vi "PinholesRolling.vi"(4 "Current Threshold [nA]":dbl, 5 "settling\ndelay":i32) -> (1 "excluded channels":i32[](array[numeric]), 2 "Current [nA]":dbl[](array[numeric]), 3 "Flag":i32[](array[numeric]))   [LabVIEW 2019]
uses:
  general_VIs/globals/QC_MeasurementSetup.vi
  InstrControl/Switching/Switching.lvclass
  InstrControl/SupplyControl/SupplyControl.lvclass
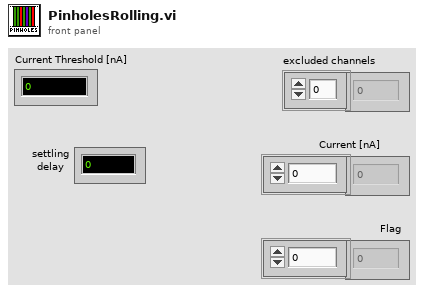
[diagram p1: front panel]
types:
  T1 = enum16{"Reference measurement", "Baseline correcetion 10V", "Baseline correcetion 100V", "Nothing"}
  T2 = cluster{"Bias Supply":refnum<class "SupplyControl.lvclass">, "SMU":refnum<class "SupplyControl.lvclass">, "LCR":refnum<class "LCRControl.lvclass">, "Probe Card Channels":i32, "Bias Voltage [V]":dbl, "First strip":i32, "Last strip":i32, "Base Voltage [V]":dbl, "Base Ramp Step [V]":dbl, "Base Ramp Interval [ms]":u32, "High Voltage [V]":dbl, "High Ramp Step [V]":dbl, "High Ramp Interval [ms]":u32, "AC frequency [Hz]":i32, "AC amplitude [V]":dbl, "RC Configuration":u16, "Single Needle":bool, "Temperature Readout":enum16{"Read Arduino", "Enter manually"}, "Arduino":refnum<class "ArduinoControl.lvclass">, "Fraction of good strips [%]":dbl, "ProbeStation":refnum<class "ProbeStationControl.lvclass">, "Switching":refnum<class "Switching.lvclass">, "Matrix used?":bool, "Matrix X Channels":cluster{"Bias Supply / SMU LO":i32, "Bias Supply / SMU HI":i32, "CV Box LO":i32, "CV Box HI":i32, "CV Box LO IN":i32, "CV Box HI IN":i32, "Volt meter LO":i32, "Volt meter HI":i32, "Mux1 C1":i32, "Mux1 C2":i32, "Mux2 C1":i32, "Mux2 C2":i32}, "Pinholes Y/N":bool, "Capacitance Y/N":bool, "Resistance Y/N":bool, "Bias Supply Name":string, "SMU Name":string, "LCR Name":string}
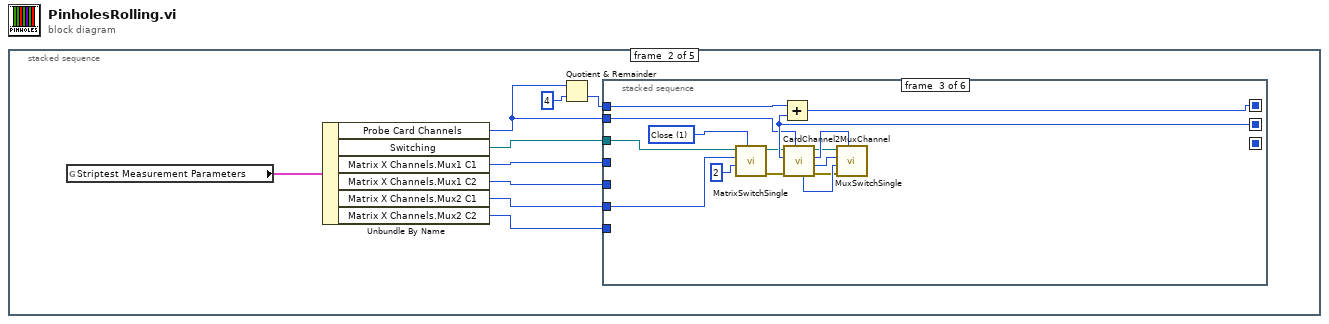
[diagram p0: block diagram]
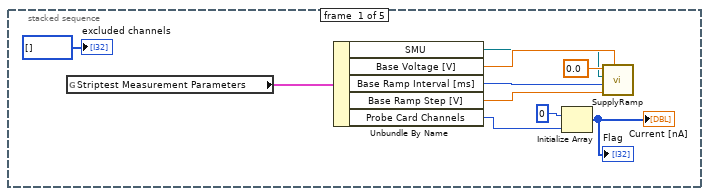
[diagram p2: hidden frame]
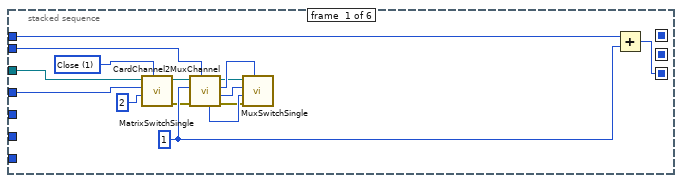
[diagram p3: hidden frame]
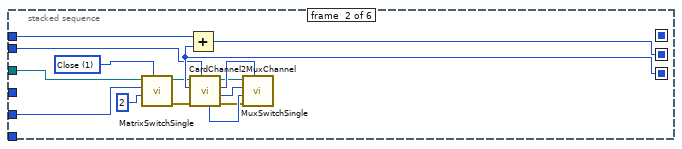
[diagram p4: hidden frame]
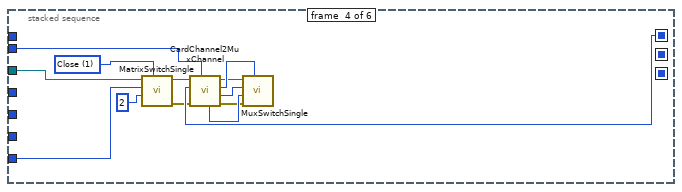
[diagram p5: hidden frame]
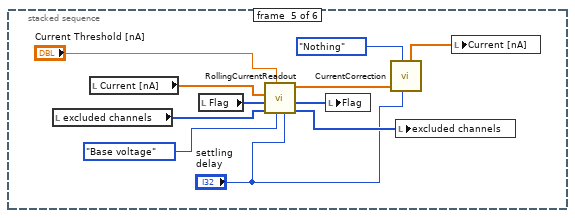
[diagram p6: hidden frame]
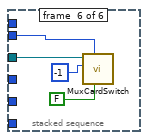
[diagram p7: hidden frame]
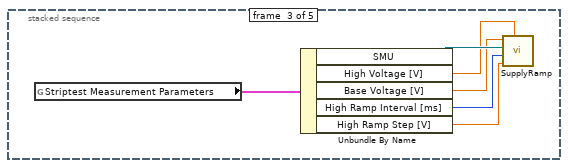
[diagram p8: hidden frame]
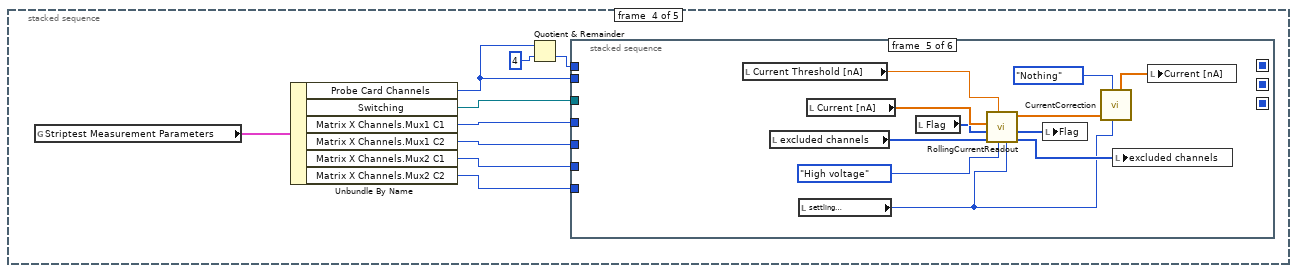
[diagram p9: hidden frame]
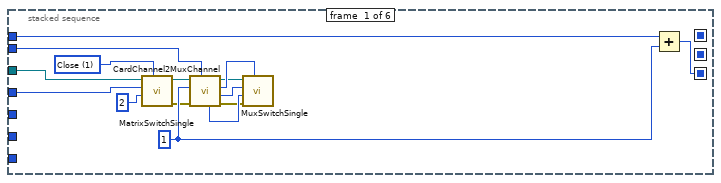
[diagram p10: hidden frame]
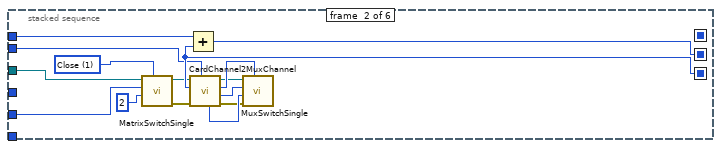
[diagram p11: hidden frame]
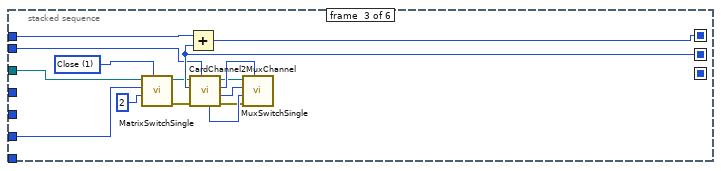
[diagram p12: hidden frame]
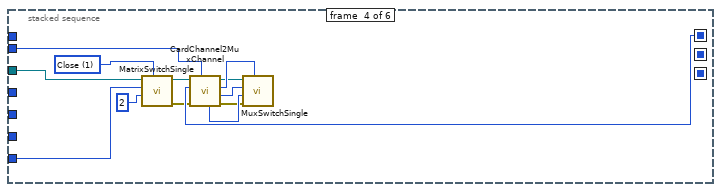
[diagram p13: hidden frame]
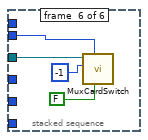
[diagram p14: hidden frame]
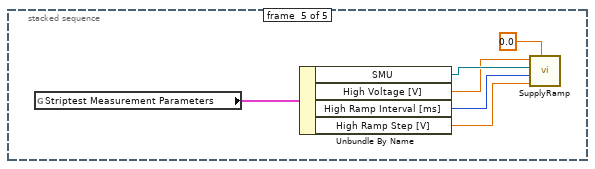
[diagram p15: hidden frame]
diagram:
  n1 = stacked-sequence {
    frame #0 {
      n2 = global read "QC_MeasurementSetup.vi" "Striptest Measurement Parameters"() -> (w6:T2)
      n3 = Unbundle By Name(w6) -> ("SMU"=w2:refnum<class "SupplyControl.lvclass">, "Base Voltage [V]"=w5:dbl, "Base Ramp Interval [ms]"=w4:u32, "Base Ramp Step [V]"=w3:dbl, "Probe Card Channels"=w1:i32)
      n4 = Initialize Array(0, w1) -> (→"Flag" →"Current [nA]":i32[])
      n5 = call "SupplyRamp.vi"("Requested Voltage"=w5, "Step Size"=w3, "Step Delay"=w4, "Supply IN"=w2, "Starting Voltage"=0.0) -> ()  [unwired: 3 in, 4 out]
      "excluded channels" <- i32[] []
    }
    frame #1 {
      n6 = global read "QC_MeasurementSetup.vi" "Striptest Measurement Parameters"() -> (w12:T2)
      n7 = Unbundle By Name(w12) -> ("Probe Card Channels"=w11:i32, "Switching"=w13:refnum<class "Switching.lvclass">, "Matrix X Channels.Mux1 C1"=w17:i32, "Matrix X Channels.Mux1 C2"=w16:i32, "Matrix X Channels.Mux2 C1"=w15:i32, "Matrix X Channels.Mux2 C2"=w14:i32)
      n8 = Quotient & Remainder(x=w11, y=4) -> (floor(x/y)=w18:i32)  [unwired: 1 out]
      n9 = stacked-sequence {
        seq-local: [w27 _ _ _ _ _] -> [_ w44 _ _ _ _]
        seq-local: [_ w43 _ _ _ _] -> [_ _ w58 _ _ _]
        seq-local: [_ _ w59 _ _ _] -> [_ _ _ w72 _ _]
        tunnel: w18 -> [w28 w36 w51 _ _ _]
        tunnel: w17 -> [w26 _ _ _ _ _]
        tunnel: w13 -> [w25 w37 w52 w66 _ w91]
        tunnel: w16 -> [_ w42 _ _ _ _]
        tunnel: w15 -> [_ _ w57 _ _ _]
        tunnel: w14 -> [_ _ _ w71 _ _]
        tunnel: w11 -> [w20 w35 w50 w65 _ w90]
        frame #0 {
          w29 = 1
          w34 = u16 1 items=["Open", "Close"] ("Switch action")
          n10 = call-dynamic "MatrixSwitchSingle.vi"("Switch action"=w34, "Matrix Y"=2, "Matrix X"=w26, "Switching in"=w25) -> ("error out"=w23:errorcluster, "Switching out"=w21:refnum<class "Switching.lvclass">)  [unwired: 5 in, 1 out]
          n11 = call-dynamic "CardChannel2MuxChannel.vi"("Probe Card Channels"=w20, "error in (no error)"=w23, "Probecard Channel No."=w29, "Switching in"=w21) -> ("error out"=w24:errorcluster, "C1 / C2"=w32:i32, "Mux No.:"=w31:u32, "Switching out"=w22:refnum<class "Switching.lvclass">, "Channel"=w33:i32)  [unwired: 2 in, 1 out]
          n12 = call-dynamic "MuxSwitchSingle.vi"("MUX address"=w31, "error in (no error)"=w24, "Channel"=w33, "C1 / C2"=w32, "Switching in"=w22) -> ()  [unwired: 4 in, 3 out]
          n13 = Add(x=w28, y=w29) -> (x+y=w27:i32)
        }
        frame #1 {
          w46 = u16 1 items=["Open", "Close"] ("Switch action")
          n14 = call-dynamic "MatrixSwitchSingle.vi"("Switch action"=w46, "Matrix Y"=2, "Matrix X"=w42, "Switching in"=w37) -> ("error out"=w39:errorcluster, "Switching out"=w38:refnum<class "Switching.lvclass">)  [unwired: 5 in, 1 out]
          n15 = Add(x=w36, y=w44) -> (x+y=w43:i32)
          n16 = call-dynamic "CardChannel2MuxChannel.vi"("Probe Card Channels"=w35, "error in (no error)"=w39, "Probecard Channel No."=w44, "Switching in"=w38) -> ("error out"=w40:errorcluster, "C1 / C2"=w48:i32, "Mux No.:"=w47:u32, "Switching out"=w41:refnum<class "Switching.lvclass">, "Channel"=w49:i32)  [unwired: 2 in, 1 out]
          n17 = call-dynamic "MuxSwitchSingle.vi"("MUX address"=w47, "error in (no error)"=w40, "Channel"=w49, "C1 / C2"=w48, "Switching in"=w41) -> ()  [unwired: 4 in, 3 out]
        }
        frame #2 {
          w63 = u16 1 items=["Open", "Close"] ("Switch action")
          n18 = call-dynamic "MatrixSwitchSingle.vi"("Switch action"=w63, "Matrix Y"=2, "Matrix X"=w57, "Switching in"=w52) -> ("error out"=w56:errorcluster, "Switching out"=w55:refnum<class "Switching.lvclass">)  [unwired: 5 in, 1 out]
          n19 = Add(x=w51, y=w58) -> (x+y=w59:i32)
          n20 = call-dynamic "CardChannel2MuxChannel.vi"("Probe Card Channels"=w50, "error in (no error)"=w56, "Probecard Channel No."=w58, "Switching in"=w55) -> ("error out"=w53:errorcluster, "C1 / C2"=w61:i32, "Mux No.:"=w62:u32, "Switching out"=w54:refnum<class "Switching.lvclass">, "Channel"=w60:i32)  [unwired: 2 in, 1 out]
          n21 = call-dynamic "MuxSwitchSingle.vi"("MUX address"=w62, "error in (no error)"=w53, "Channel"=w60, "C1 / C2"=w61, "Switching in"=w54) -> ()  [unwired: 4 in, 3 out]
        }
        frame #3 {
          w74 = u16 1 items=["Open", "Close"] ("Switch action")
          n22 = call-dynamic "MatrixSwitchSingle.vi"("Switch action"=w74, "Matrix Y"=2, "Matrix X"=w71, "Switching in"=w66) -> ("error out"=w68:errorcluster, "Switching out"=w70:refnum<class "Switching.lvclass">)  [unwired: 5 in, 1 out]
          n23 = call-dynamic "CardChannel2MuxChannel.vi"("Probe Card Channels"=w65, "error in (no error)"=w68, "Probecard Channel No."=w72, "Switching in"=w70) -> ("error out"=w67:errorcluster, "C1 / C2"=w76:i32, "Mux No.:"=w75:u32, "Switching out"=w69:refnum<class "Switching.lvclass">, "Channel"=w77:i32)  [unwired: 2 in, 1 out]
          n24 = call-dynamic "MuxSwitchSingle.vi"("MUX address"=w75, "error in (no error)"=w67, "Channel"=w77, "C1 / C2"=w76, "Switching in"=w69) -> ()  [unwired: 4 in, 3 out]
        }
        frame #4 {
          n25 = local read "excluded channels"() -> (w86:i32[])
          n26 = local read "Current [nA]"() -> (w87:dbl[])
          n27 = local read "Flag"() -> (w85:i32[])
          n28 = call "RollingCurrentReadout.vi"("settling\ndelay"="settling\ndelay", "Base/High Voltage?"=enum16{"Base voltage", "High voltage"}."Base voltage", "Current Threshold [nA]"="Current Threshold [nA]", "disabled channels IN"=w86, "Flag IN"=w85, "Current Array IN [nA]"=w87) -> ("disabled channels OUT"=w84:i32[], "Flag OUT"=w83:i32[], "Current Array OUT [nA]"=w82:dbl[])  [unwired: 2 in, 1 out]
          n29 = local write "Flag"(w83) -> ()
          n30 = call "CurrentCorrection.vi"("Action"=T1."Nothing", "Current IN"=w82, "settling\ndelay"="settling\ndelay") -> ("Current OUT"=w81:dbl[])  [unwired: 2 in, 4 out]
          n31 = local write "excluded channels"(w84) -> ()
          n32 = local write "Current [nA]"(w81) -> ()
        }
        frame #5 {
          n33 = call-dynamic "MuxCardSwitch.vi"("Single Needle"=FALSE, "Probe Card Channels"=w90, "Switch to channel"=-1, "Switching in"=w91) -> ()  [unwired: 5 in, 3 out]
        }
      }
    }
    frame #2 {
      n34 = global read "QC_MeasurementSetup.vi" "Striptest Measurement Parameters"() -> (w98:T2)
      n35 = Unbundle By Name(w98) -> ("SMU"=w95:refnum<class "SupplyControl.lvclass">, "High Voltage [V]"=w93:dbl, "Base Voltage [V]"=w94:dbl, "High Ramp Interval [ms]"=w96:u32, "High Ramp Step [V]"=w97:dbl)
      n36 = call "SupplyRamp.vi"("Requested Voltage"=w93, "Step Size"=w97, "Step Delay"=w96, "Supply IN"=w95, "Starting Voltage"=w94) -> ()  [unwired: 3 in, 4 out]
    }
    frame #3 {
      n37 = global read "QC_MeasurementSetup.vi" "Striptest Measurement Parameters"() -> (w100:T2)
      n38 = Unbundle By Name(w100) -> ("Probe Card Channels"=w99:i32, "Switching"=w105:refnum<class "Switching.lvclass">, "Matrix X Channels.Mux1 C1"=w104:i32, "Matrix X Channels.Mux1 C2"=w103:i32, "Matrix X Channels.Mux2 C1"=w102:i32, "Matrix X Channels.Mux2 C2"=w101:i32)
      n39 = Quotient & Remainder(x=w99, y=4) -> (floor(x/y)=w106:i32)  [unwired: 1 out]
      n40 = stacked-sequence {
        seq-local: [w115 _ _ _ _ _] -> [_ w132 _ _ _ _]
        seq-local: [_ w131 _ _ _ _] -> [_ _ w147 _ _ _]
        seq-local: [_ _ w146 _ _ _] -> [_ _ _ w160 _ _]
        tunnel: w106 -> [w117 w124 w139 _ _ _]
        tunnel: w105 -> [w114 w125 w140 w154 _ w178]
        tunnel: w104 -> [w113 _ _ _ _ _]
        tunnel: w99 -> [w108 w123 w138 w153 _ w177]
        tunnel: w103 -> [_ w130 _ _ _ _]
        tunnel: w102 -> [_ _ w145 _ _ _]
        tunnel: w101 -> [_ _ _ w159 _ _]
        frame #0 {
          w116 = 1
          w122 = u16 1 items=["Open", "Close"] ("Switch action")
          n41 = call-dynamic "MatrixSwitchSingle.vi"("Switch action"=w122, "Matrix Y"=2, "Matrix X"=w113, "Switching in"=w114) -> ("error out"=w110:errorcluster, "Switching out"=w112:refnum<class "Switching.lvclass">)  [unwired: 5 in, 1 out]
          n42 = call-dynamic "CardChannel2MuxChannel.vi"("Probe Card Channels"=w108, "error in (no error)"=w110, "Probecard Channel No."=w116, "Switching in"=w112) -> ("error out"=w109:errorcluster, "C1 / C2"=w120:i32, "Mux No.:"=w119:u32, "Switching out"=w111:refnum<class "Switching.lvclass">, "Channel"=w121:i32)  [unwired: 2 in, 1 out]
          n43 = call-dynamic "MuxSwitchSingle.vi"("MUX address"=w119, "error in (no error)"=w109, "Channel"=w121, "C1 / C2"=w120, "Switching in"=w111) -> ()  [unwired: 4 in, 3 out]
          n44 = Add(x=w117, y=w116) -> (x+y=w115:i32)
        }
        frame #1 {
          w134 = u16 1 items=["Open", "Close"] ("Switch action")
          n45 = call-dynamic "MatrixSwitchSingle.vi"("Switch action"=w134, "Matrix Y"=2, "Matrix X"=w130, "Switching in"=w125) -> ("error out"=w129:errorcluster, "Switching out"=w128:refnum<class "Switching.lvclass">)  [unwired: 5 in, 1 out]
          n46 = Add(x=w124, y=w132) -> (x+y=w131:i32)
          n47 = call-dynamic "CardChannel2MuxChannel.vi"("Probe Card Channels"=w123, "error in (no error)"=w129, "Probecard Channel No."=w132, "Switching in"=w128) -> ("error out"=w127:errorcluster, "C1 / C2"=w136:i32, "Mux No.:"=w135:u32, "Switching out"=w126:refnum<class "Switching.lvclass">, "Channel"=w137:i32)  [unwired: 2 in, 1 out]
          n48 = call-dynamic "MuxSwitchSingle.vi"("MUX address"=w135, "error in (no error)"=w127, "Channel"=w137, "C1 / C2"=w136, "Switching in"=w126) -> ()  [unwired: 4 in, 3 out]
        }
        frame #2 {
          w151 = u16 1 items=["Open", "Close"] ("Switch action")
          n49 = call-dynamic "MatrixSwitchSingle.vi"("Switch action"=w151, "Matrix Y"=2, "Matrix X"=w145, "Switching in"=w140) -> ("error out"=w144:errorcluster, "Switching out"=w141:refnum<class "Switching.lvclass">)  [unwired: 5 in, 1 out]
          n50 = Add(x=w139, y=w147) -> (x+y=w146:i32)
          n51 = call-dynamic "CardChannel2MuxChannel.vi"("Probe Card Channels"=w138, "error in (no error)"=w144, "Probecard Channel No."=w147, "Switching in"=w141) -> ("error out"=w143:errorcluster, "C1 / C2"=w149:i32, "Mux No.:"=w150:u32, "Switching out"=w142:refnum<class "Switching.lvclass">, "Channel"=w148:i32)  [unwired: 2 in, 1 out]
          n52 = call-dynamic "MuxSwitchSingle.vi"("MUX address"=w150, "error in (no error)"=w143, "Channel"=w148, "C1 / C2"=w149, "Switching in"=w142) -> ()  [unwired: 4 in, 3 out]
        }
        frame #3 {
          w162 = u16 1 items=["Open", "Close"] ("Switch action")
          n53 = call-dynamic "MatrixSwitchSingle.vi"("Switch action"=w162, "Matrix Y"=2, "Matrix X"=w159, "Switching in"=w154) -> ("error out"=w158:errorcluster, "Switching out"=w155:refnum<class "Switching.lvclass">)  [unwired: 5 in, 1 out]
          n54 = call-dynamic "CardChannel2MuxChannel.vi"("Probe Card Channels"=w153, "error in (no error)"=w158, "Probecard Channel No."=w160, "Switching in"=w155) -> ("error out"=w157:errorcluster, "C1 / C2"=w164:i32, "Mux No.:"=w163:u32, "Switching out"=w156:refnum<class "Switching.lvclass">, "Channel"=w165:i32)  [unwired: 2 in, 1 out]
          n55 = call-dynamic "MuxSwitchSingle.vi"("MUX address"=w163, "error in (no error)"=w157, "Channel"=w165, "C1 / C2"=w164, "Switching in"=w156) -> ()  [unwired: 4 in, 3 out]
        }
        frame #4 {
          n56 = local read "Current Threshold [nA]"() -> (w171:dbl)
          n57 = local read "excluded channels"() -> (w175:i32[])
          n58 = local read "settling\ndelay"() -> (w167:i32)
          n59 = local read "Current [nA]"() -> (w176:dbl[])
          n60 = local read "Flag"() -> (w174:i32[])
          n61 = call "RollingCurrentReadout.vi"("settling\ndelay"=w167, "Base/High Voltage?"=enum16{"Base voltage", "High voltage"}."High voltage", "Current Threshold [nA]"=w171, "disabled channels IN"=w175, "Flag IN"=w174, "Current Array IN [nA]"=w176) -> ("disabled channels OUT"=w173:i32[], "Flag OUT"=w172:i32[], "Current Array OUT [nA]"=w170:dbl[])  [unwired: 2 in, 1 out]
          n62 = local write "Flag"(w172) -> ()
          n63 = call "CurrentCorrection.vi"("Action"=T1."Nothing", "Current IN"=w170, "settling\ndelay"=w167) -> ("Current OUT"=w169:dbl[])  [unwired: 2 in, 4 out]
          n64 = local write "excluded channels"(w173) -> ()
          n65 = local write "Current [nA]"(w169) -> ()
        }
        frame #5 {
          n66 = call-dynamic "MuxCardSwitch.vi"("Single Needle"=FALSE, "Probe Card Channels"=w177, "Switch to channel"=-1, "Switching in"=w178) -> ()  [unwired: 5 in, 3 out]
        }
      }
    }
    frame #4 {
      n67 = global read "QC_MeasurementSetup.vi" "Striptest Measurement Parameters"() -> (w185:T2)
      n68 = Unbundle By Name(w185) -> ("SMU"=w184:refnum<class "SupplyControl.lvclass">, "High Voltage [V]"=w181:dbl, "High Ramp Interval [ms]"=w182:u32, "High Ramp Step [V]"=w183:dbl)
      n69 = call "SupplyRamp.vi"("Requested Voltage"=0.0, "Step Size"=w183, "Step Delay"=w182, "Supply IN"=w184, "Starting Voltage"=w181) -> ()  [unwired: 3 in, 4 out]
    }
  }
